vi "ITU_Frequency.vi"(11 "Frequency":dbl) -> (3 "ITU_468":dbl)   [LabVIEW 2015]
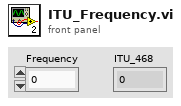
[diagram p1: front panel]
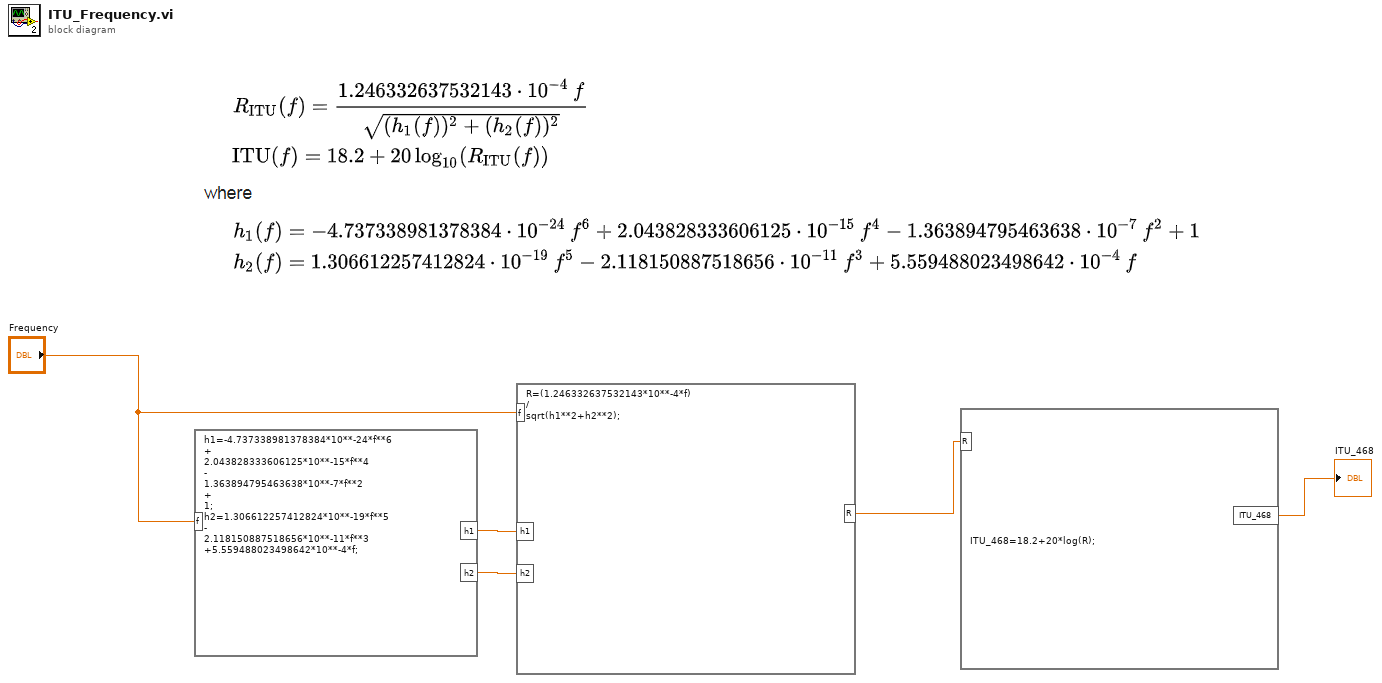
[diagram p0: block diagram]
diagram:
  n1 = formula code="h1=-4.737338981378384*10**-24*f**6\n+\n2.043828333606125*10**-15*f**4\n-\n1.363894795463638*10**-7*f**2\n+\n1;\nh2=1.306612257412824*10**-19*f**5\n-\n2.118150887518656*10**-11*f**3\n+5.559488023498642*10**-4*f;"("f"="Frequency") -> ("h1"=w2:dbl, "h2"=w3:dbl)
  n2 = formula code="R=(1.246332637532143*10**-4*f)\n/\nsqrt(h1**2+h2**2);"("h1"=w2, "h2"=w3, "f"="Frequency") -> ("R"=w4:dbl)
  n3 = formula code="ITU_468=18.2+20*log(R);"("R"=w4) -> ("ITU_468"=→"ITU_468":dbl)
